vi "Wave2D_Init Data_Coef Mtrx.vi"(8 "BC start index":i32, 9 "length":i32, 10 "ks":dbl, 11 "Boundary Condition":cluster{"type":T4, "Value":dbl[][]}[](array[cluster]) {"type" items=["Dirichlet", "Neumann"]}) -> (0 "error":i32, 2 "LU of A":T1, 3 "A":T3)   [LabVIEW 2017, in "NI_PDE.lvlib"]
uses:
  <vilib>/gmath/NI_PDE.lvlib
  <vilib>/gmath/pde.llb/Common/PDE_BC Type.ctl
  <vilib>/Analysis/Matrix/Datatypes/RealMatrix.ctl
  <vilib>/Analysis/Matrix/NI_Matrix.lvlib
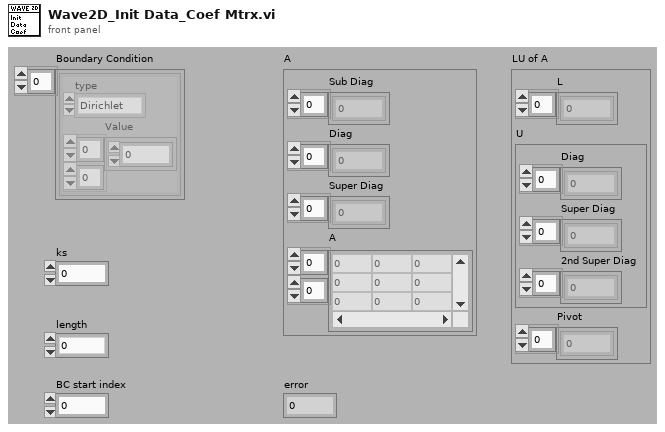
[diagram p1: front panel]
types:
  T1 = cluster{"L":dbl[], "U":cluster{"Diag":dbl[], "Super Diag":dbl[], "2nd Super Diag":dbl[]}, "Pivot":i32[]}
  T2 = typedef "NI_Matrix.lvlib/RealMatrix.ctl" = dbl[][]
  T3 = cluster{"Sub Diag":dbl[], "Diag":dbl[], "Super Diag":dbl[], "A":T2}
  T4 = typedef "NI_PDE.lvlib/PDE_BC Type.ctl" = i32
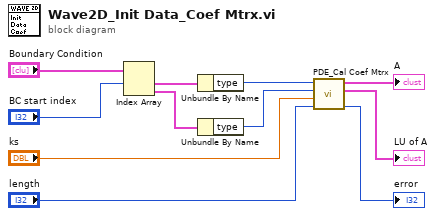
[diagram p0: block diagram]
diagram:
  n1 = Index Array(array="Boundary Condition", index #1="BC start index") -> (element #1=w10:cluster{"type":T4, "Value":dbl[][]}, element #2=w9:cluster{"type":T4, "Value":dbl[][]})  [unwired: 1 in]
  n2 = Unbundle By Name(w10) -> ("type"=w7:T4)
  n3 = Unbundle By Name(w9) -> ("type"=w6:T4)
  n4 = call <vilib>:"PDE_Cal Coef Mtrx.vi"("length"="length", "ks"="ks", "end type"=w6, "start type"=w7) -> ("error"=→"error":i32, "LU of A"=→"LU of A":T1, "A"=→"A":T3)  [unwired: 5 out]
